vi "Query Remote Trace Connection Count.vi"(8 "error in (no error)":errorcluster, 11 "VISA resource name":refnum<visa-resource-name>) -> (0 "error out":errorcluster, 1 "Max Connections":i32, 2 "Open Connections":i32, 3 "VISA resource name out":refnum<visa-resource-name>)   [LabVIEW 2020, in "Rohde&Schwarz CMXP Base.lvlib"]
doc: "Queries the number of remote control connections.\n\nAttribute:\n-\n\nRemote-control command:\nFETCh:BASE:RTRace:CONNections:COUNt?"
uses:
  <instrlib>/Rohde&Schwarz CMXP Base/Rohde&Schwarz CMXP Base.lvlib
  <instrlib>/Rohde&Schwarz CMXP Base/Private/rsidr_core.llb/rsidr_core.lvlib
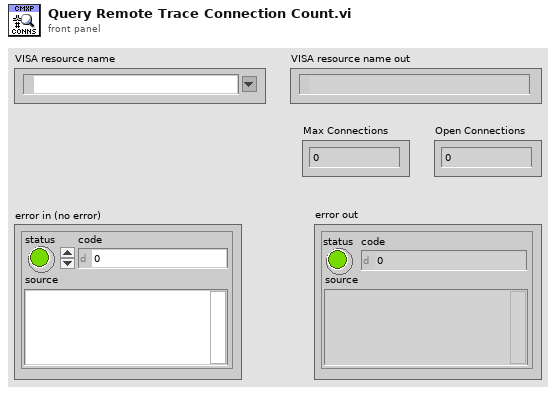
[diagram p1: front panel]
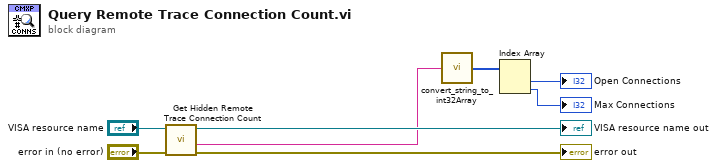
[diagram p0: block diagram]
diagram:
  n1 = call "Get Hidden Remote Trace Connection Count"("error in (no error)"="error in (no error)", "instrument handle"="VISA resource name") -> ("error out"=→"error out":errorcluster, "Hidden Remote Trace Connection Count"=w1:string, "instrument handle out"=→"VISA resource name out":refnum<visa-resource-name>)  [unwired: 7 in]
  n2 = call <instrlib>:"convert_string_to_int32Array.vi"("string in"=w1) -> ("int32 array out"=w6:i32[])  [unwired: 3 in, 1 out]
  n3 = Index Array(array=w6) -> (element #1=→"Open Connections":i32, element #2=→"Max Connections":i32)  [unwired: 2 in]
